vi "Write_TDMS.vi"() -> ()   [LabVIEW 2018]
uses:
  <vilib>/measure/NI_MABase.lvlib
panel:
  out "웨이브폼 차트 2":waveform(dbl)(graph)
  out "웨이브폼 차트":waveform(dbl)(graph)
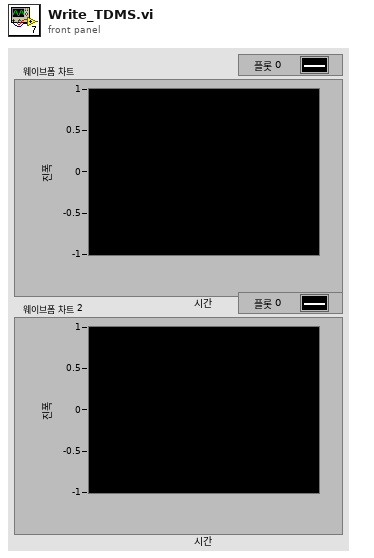
[diagram p1: front panel]
types:
  T1 = enum16{"Sine Wave", "Triangle Wave", "Square Wave", "Sawtooth Wave"}
  T2 = enum16{"open", "open or create", "create or replace", "create", "open (read-only)"}
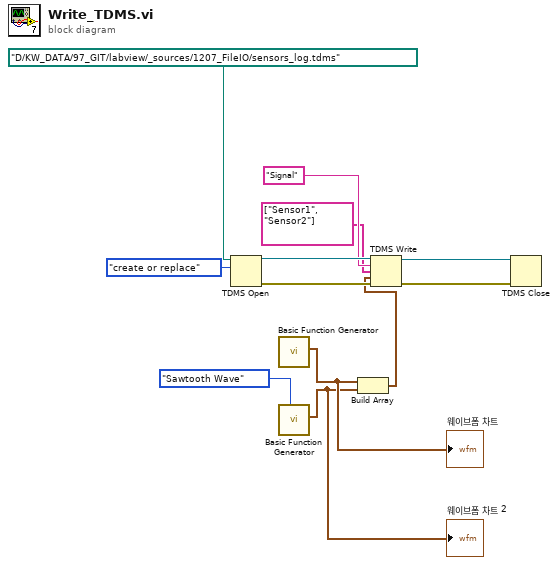
[diagram p0: block diagram]
diagram:
  n1 = TDMS Open(10:T2."create or replace" ("동작(0:open)"), 11:path "D:/KW_DATA/97_GIT/labview/_sources/1207_FileIO/sensors_log.tdms" ("파일 경로")) -> (0:w11:errorcluster, 3:w12:refnum<k34>)  [unwired: 5 in]
  n2 = call <vilib>:"Basic Function Generator.vi"() -> ("signal out"=w2:waveform(dbl))  [unwired: 9 in, 2 out]
  "웨이브폼 차트" <- w2
  n3 = call <vilib>:"Basic Function Generator.vi"("signal type"=T1."Sawtooth Wave") -> ("signal out"=w1:waveform(dbl))  [unwired: 8 in, 2 out]
  "웨이브폼 차트 2" <- w1
  n4 = Build Array(w2, w1) -> (w5:waveform(dbl)[])
  n5 = TDMS Write(0:w12, 5:"Signal" ("그룹 이름 입력(제목없음)"), 7:string[] ["Sensor1", "Sensor2"] ("채널 이름 입력(제목없음)"), 9:w5, 11:w11) -> (4:w10:refnum<k34>, 15:w9:errorcluster)  [unwired: 1 in, 2 out]
  n6 = TDMS Close(8:w9, 11:w10) -> ()  [unwired: 2 out]
